vi "Irradiance Panel 1006 - run only.vi"(9 "Boolean":bool) -> (8 "Irradiance":dbl)   [LabVIEW 2021]
uses:
  irradiance 1018_global variable.vi
panel:
  in  "Pyranometer sensitivity (µV/W/m²) 2":dbl=7.02e-05
  out "Pyranometer":dbl(graph)
  in  "Measurements per channel 2":i32=3 min=1 max=1000
  in  "Measurement channels 2":string="1006"
  out "error save file":errorcluster
  in  "VISA resource name":refnum<visa-resource-name>="USB0::2391::1287::MY44008368::0::INSTR"
  in  "error in (no error)":errorcluster
  out "VISA/Instrument Errors":errorcluster
  # "TO DO\n- automatically update date at every reading\n- append new reading to the same file\n- take mean of multiple readings"
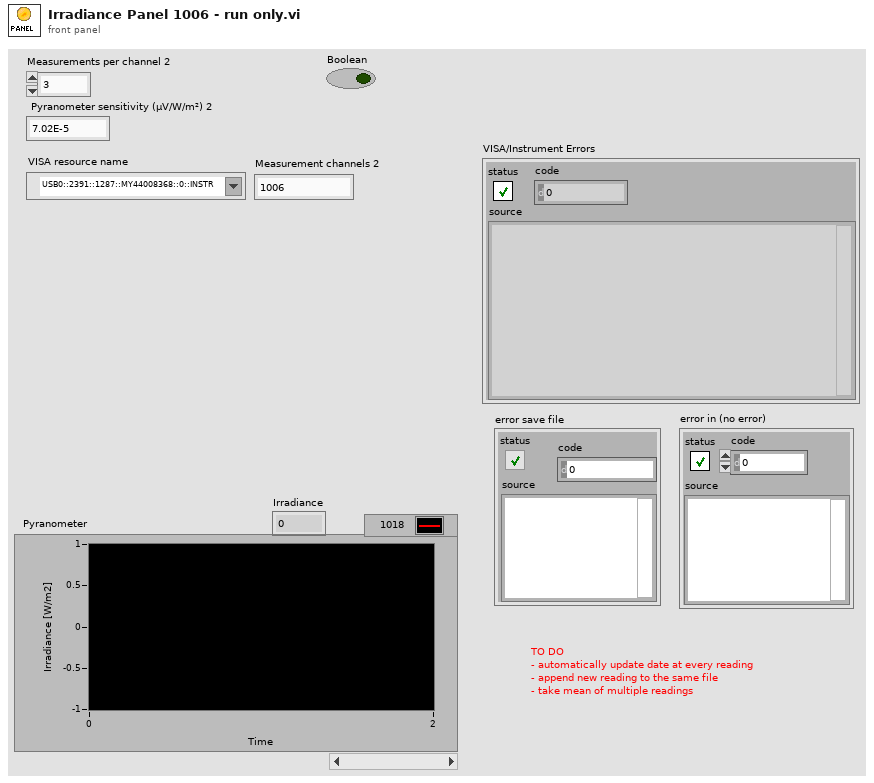
[diagram p1: front panel]
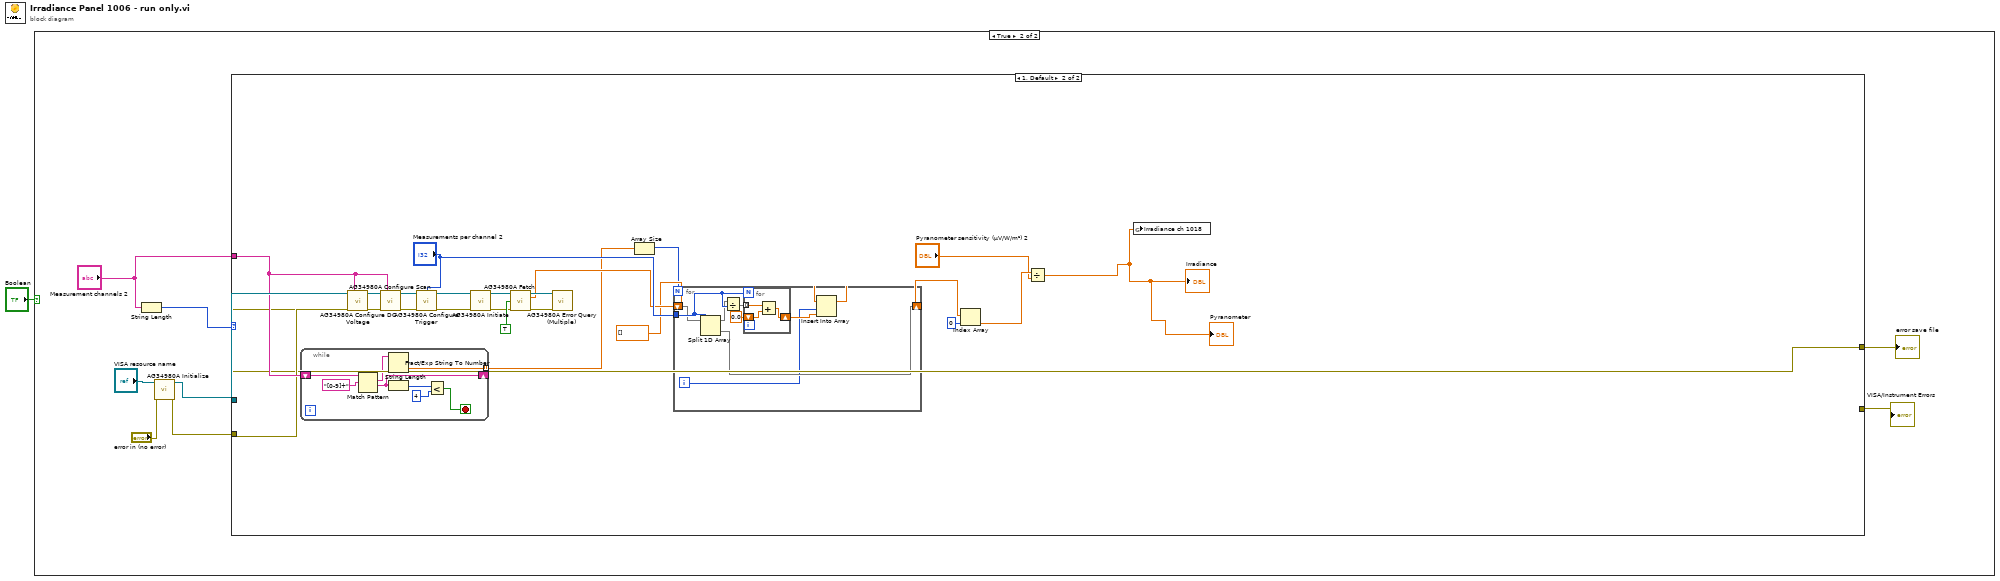
[diagram p0: block diagram]
diagram:
  n1 = case shown="True" "Boolean" {
    frame False {
    }
    frame True {
      n2 = String Length(string="Measurement channels 2") -> (length=w4:i32)
      n3 = call "AG34980A Initialize.vi"("VISA resource name"="VISA resource name", "error in (no error)"="error in (no error)") -> ("VISA session"=w3:refnum<visa-resource-name>, "error out"=w2:errorcluster)  [unwired: 12 in]
      n4 = case shown="1, Default" w4 {
        tunnel: [w10 _] -> w9
        tunnel: w3 -> [_ w35]
        tunnel: [_ w11] -> w6
        tunnel: "Measurement channels 2" -> [_ w34]
        tunnel: w2 -> [w10 w13]
        frame 0 {
        }
        frame 1, Default {
          n5 = while {
            shift-right: [w49] -> _
            shift-left: w34 -> [w52]
            tunnel: [w51] -> w18 mode=indexing
            stop <- w50 stop-if-true
            n6 = Match Pattern(string=w52, regular expression="[0-9]+" ("Thermocouple channels")) -> (match substring=w56:string, after substring=w49:string)  [unwired: 1 in, 2 out]
            n7 = Fract/Exp String To Number(string=w56) -> (number=w51:dbl)  [unwired: 3 in, 1 out]
            n8 = String Length(string=w49) -> (length=w54:i32)
            n9 = Less?(x=w54, y=4) -> (x < y?=w50:bool)
          }
          n10 = call "AG34980A Configure DC Voltage.vi"("VISA resource name"=w35, "Channel List(empty)"=w34, "error in (no error)"=w13) -> ("VISA resource name out"=w33:refnum<visa-resource-name>, "error out"=w27:errorcluster)  [unwired: 11 in]
          n11 = call "AG34980A Configure Scan.vi"("VISA resource name"=w33, "Scan List(empty)"=w34, "error in (no error)"=w27) -> ("VISA resource name out"=w32:refnum<visa-resource-name>, "error out"=w26:errorcluster)  [unwired: 11 in]
          n12 = call "AG34980A Configure Trigger.vi"("VISA resource name"=w32, "Sample Count (1)"="Measurements per channel 2", "error in (no error)"=w26) -> ("VISA resource name out"=w31:refnum<visa-resource-name>, "error out"=w25:errorcluster)  [unwired: 11 in]
          n13 = call "AG34980A Initiate.vi"("VISA resource name"=w31, "error in (no error)"=w25) -> ("VISA resource name out"=w30:refnum<visa-resource-name>, "error out"=w24:errorcluster)  [unwired: 12 in]
          n14 = call "AG34980A Fetch.vi"("VISA resource name"=w30, "Numbers Only (T:On)"=TRUE, "error in (no error)"=w24) -> ("VISA resource name out"=w29:refnum<visa-resource-name>, "Output Data (Numbers Only)"=w21:dbl[], "error out"=w23:errorcluster)  [unwired: 9 in, 1 out]
          n15 = call "AG34980A Error Query (Multiple).vi"("VISA resource name"=w29, "error in (no error)"=w23) -> ("error out"=w11:errorcluster)  [unwired: 10 in, 3 out]
          n16 = Array Size(array=w18) -> (size(s)=w19:i32)
          n17 = for {
            N: w19 -> [_]
            shift-right: [w45] -> _
            shift-left: w21 -> [w37]
            shift-right: [w39] -> w15
            shift-left: dbl[] [] -> [w40]
            tunnel: "Measurements per channel 2" -> [w38]
            i -> [w41]
            n18 = Split 1D Array(array=w37, index=w38) -> (first subarray=w36:dbl[], second subarray=w45:dbl[])
            n19 = Divide(x=w36, y=w38) -> (x/y=w43:dbl[])
            n20 = for {
              N: w38 -> [_]
              shift-right: [w46] -> w42
              shift-left: 0.0 ("index") -> [w48]
              tunnel: w43 -> [w47] mode=indexing
              n21 = Add(x=w47, y=w48) -> (x+y=w46:dbl)
            }
            n22 = Insert Into Array(array=w40, index=w41, new element=w42) -> (w39:dbl[])
          }
          n23 = Index Array(array=w15, index=0) -> (element=w16:dbl)
          n24 = Divide(x=w16, y="Pyranometer sensitivity (µV/W/m²) 2") -> (x/y=w12:dbl)
          "Pyranometer" <- w12
          "Irradiance" <- w12
          n25 = global write "irradiance 1018_global variable.vi" "Irradiance ch 1018"(w12) -> ()
        }
      }
      "VISA/Instrument Errors" <- w9
      "error save file" <- w6
    }
  }
